vi "Logging List Logs.vi"(0 "Path":path, 1 "Name":string, 2 "Remote":bool, 3 "Host":string) -> (5 "filenames":string[](array[string]))   [LabVIEW 2012, in "femtoRoboLib.lvlib"]
uses:
  femtoRoboLib.lvlib
  <vilib>/FTP/NI_FTP.lvlib
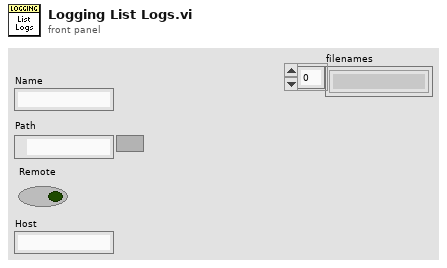
[diagram p1: front panel]
types:
  T1 = typedef "NI_FTP.lvlib/FTP Session.ctl" = refnum<k5>
  T2 = typedef "NI_FTP.lvlib/FTP File Info.ctl" = cluster{"type":enum16{"unknown", "file", "dir", "link"}, "permissions":string, "owner":string, "group":string, "size":i32, "date":string, "name":string, "link name":string}
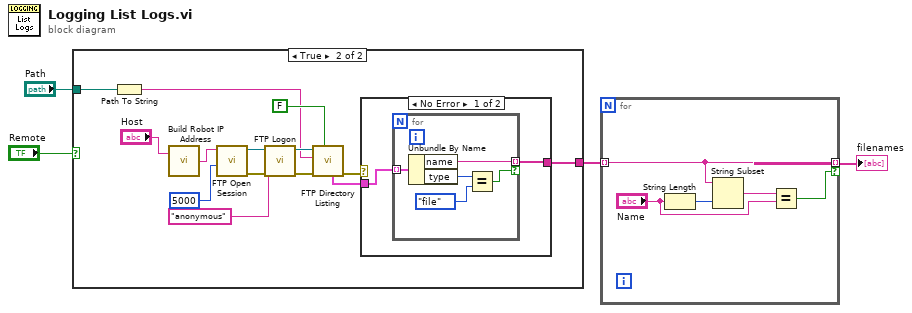
[diagram p0: block diagram]
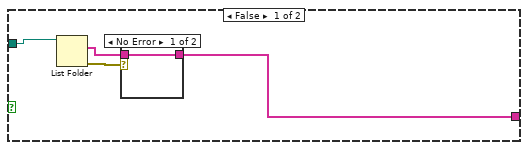
[diagram p2: hidden frame]
diagram:
  n1 = case shown="True" "Remote" {
    tunnel: "Path" -> [w5 w13]
    tunnel: [w6 w18] -> w3
    frame False {
      n2 = List Folder(path=w5) -> (filenames=w7:string[], error out=w8:errorcluster)  [unwired: 3 in, 2 out]
      n3 = case shown="No Error" w8 {
        tunnel: w7 -> [w9 _]
        tunnel: [w9 _] -> w6
        frame No Error {
        }
        frame Error {
        }
      }
    }
    frame True {
      n4 = Path To String(path=w13) -> (string=w11:string)
      n5 = call "Build Robot IP Address.vi"("In Address"="Host") -> ("Out Address"=w22:string)  [unwired: 1 in]
      n6 = call <vilib>:"FTP Open Session.vi"("timeout ms (60000)"=5000, "address"=w22) -> ("error out"=w15:errorcluster, "ftp session"=w21:T1)  [unwired: 6 in, 2 out]
      n7 = call <vilib>:"FTP Logon.vi"("error in (no error)"=w15, "user"="anonymous", "ftp session"=w21) -> ("error out"=w14:errorcluster, "ftp session out"=w17:T1)  [unwired: 5 in, 2 out]
      n8 = call <vilib>:"FTP Directory Listing.vi"("active (T)"=FALSE, "error in (no error)"=w14, "directory path"=w11, "ftp session"=w17) -> ("error out"=w16:errorcluster, "dir list"=w19:T2[])  [unwired: 3 in, 3 out]
      n9 = case shown="No Error" w16 {
        tunnel: w19 -> [w25 _]
        tunnel: [w24 _] -> w18
        frame No Error {
          n10 = for {
            tunnel: w25 -> [w30] mode=indexing
            tunnel: [w29] -> w24 mode=indexing if=w26
            n11 = Unbundle By Name(w30) -> ("name"=w29:string, "type"=w28:enum16{"unknown", "file", "dir", "link"})
            n12 = Equal?(x=w28, y=enum16{"unknown", "file", "dir", "link"}."file" ("type")) -> (x = y?=w26:bool)
          }
        }
        frame Error {
        }
      }
    }
  }
  n13 = for {
    tunnel: w3 -> [w35] mode=indexing
    tunnel: [w35] -> w2 mode=indexing if=w31
    n14 = String Length(string="Name") -> (length=w34:i32)
    n15 = String Subset(string=w35, length (rest)=w34) -> (substring=w33:string)  [unwired: 1 in]
    n16 = Equal?(x=w33, y="Name") -> (x = y?=w31:bool)
  }
  "filenames" <- w2
